vi "14_2.vi"() -> ()   [LabVIEW 2018]
uses:
  <userlib>/_OpenG.lib/dictionary/dictionary.llb/Dictionary Update (by scalar value)__ogtk.vi
panel:
  out "sum":u64
  out "Array":u64[](array[numeric])
  out "items":cluster{"key":variant, "value":variant}[](array[cluster])
  out "Mask":string[](array[string])
  out "array":string[](array[string])
  in  "Input":string
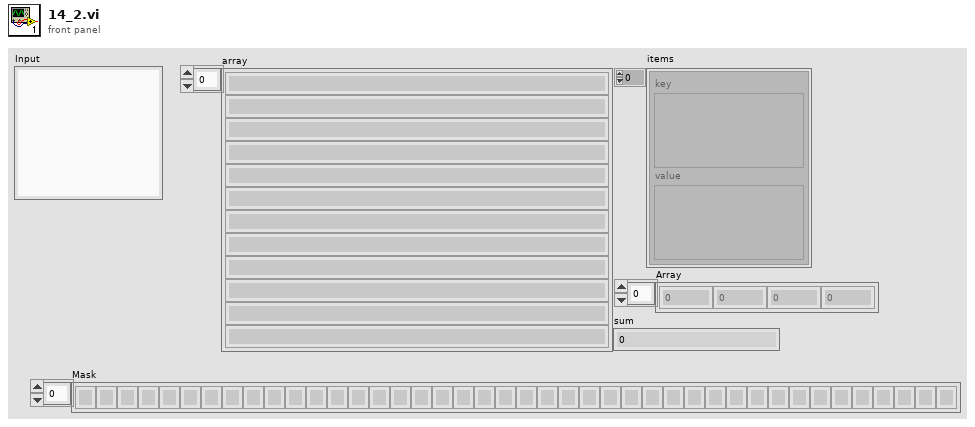
[diagram p1: front panel]
types:
  T1 = typedef "Dictionary Object RefNum__ogtk.ctl" = refnum<k1>
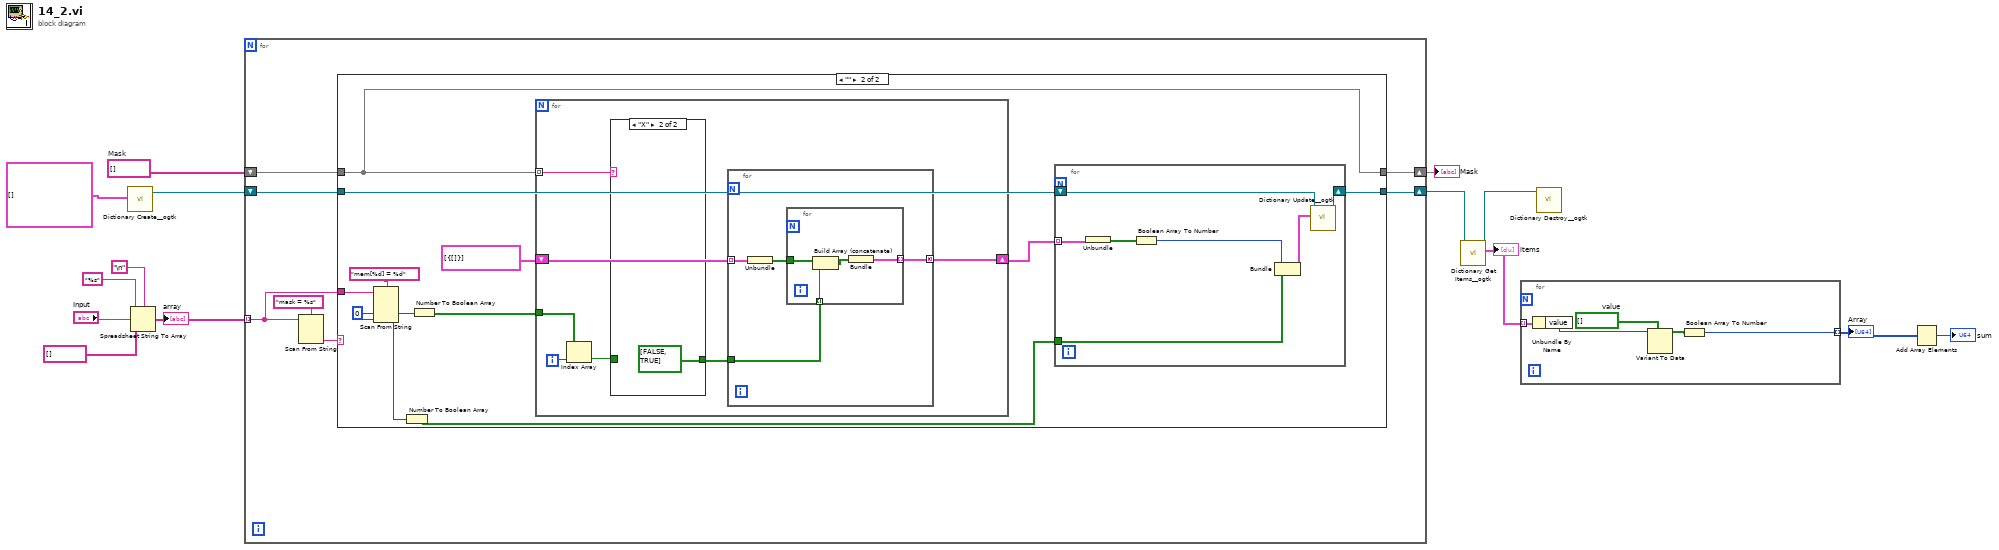
[diagram p0: block diagram]
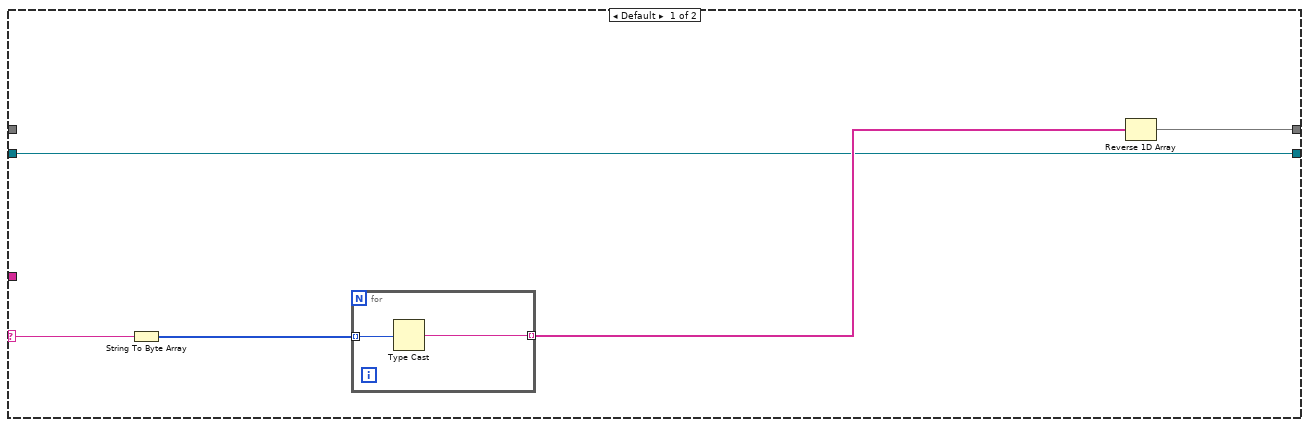
[diagram p2: hidden frame]
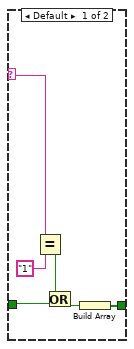
[diagram p3: hidden frame]
diagram:
  w9 = string[] []  # Mask
  n1 = call <userlib>:"Dictionary Create__ogtk.vi"("initial dictionary (empty)"=cluster{"key":u64, "value":bool[]}[] []) -> ("dictionary out"=w7:T1)  [unwired: 9 in, 1 out]
  n2 = Spreadsheet String To Array(delimiter (Tab)="\n", format string="%s", spreadsheet string="Input", array type (2D Dbl)=string[] []) -> (array=w10:string[])
  "array" <- w10
  n3 = for {
    tunnel: w10 -> [w15] mode=indexing
    shift-right: [w18] -> w8
    shift-left: w9 -> [w19]
    shift-right: [w16] -> w5
    shift-left: w7 -> [w17]
    n4 = Scan From String(format string="mask = %s", input string=w15) -> (output 1=w20:string)  [unwired: 3 in, 3 out]
    n5 = case shown="\"\"" w20 {
      selector: w20 -> [w26 _]
      tunnel: w19 -> [_ w37]
      tunnel: [w22 w37] -> w18
      tunnel: w17 -> [w23 w36]
      tunnel: [w23 w38] -> w16
      tunnel: w15 -> [_ w40]
      frame Default {
        n6 = String To Byte Array(string=w26) -> (unsigned byte array=w25:u8[])
        n7 = for {
          tunnel: w25 -> [w28] mode=indexing
          tunnel: [w27] -> w24 mode=indexing
          n8 = Type Cast(x=w28) -> (*(type *) &x=w27:string)  [unwired: 1 in]
        }
        n9 = Reverse 1D Array(array=w24) -> (reversed array=w22:string[])
      }
      frame "" {
        w33 = u64 0
        n10 = Scan From String(format string="mem[%d] = %d", input string=w40, default 1=w33, default 2=w33) -> (output 1=w32:u64, output 2=w34:u64)  [unwired: 2 in, 3 out]
        n11 = Number To Boolean Array(number=w34) -> (Boolean array=w35:bool[])
        n12 = Number To Boolean Array(number=w32) -> (Boolean array=w31:bool[])
        n13 = for {
          tunnel: w37 -> [w54] mode=indexing
          shift-right: [w48] -> w29
          shift-left: cluster{bool[]}[] [{[]}] -> [w50]
          tunnel: w31 -> [w51]
          i -> [w52]
          n14 = Index Array(array=w51, index=w52) -> (element=w53:bool)
          n15 = case shown="\"X\"" w54 {
            selector: w54 -> [w68 _]
            tunnel: [w63 bool[] [FALSE, TRUE]] -> w49
            tunnel: w53 -> [w66 _]
            frame Default {
              n16 = Equal?(x=w68, y="1") -> (x = y?=w65:bool)
              n17 = Or(x=w65, y=w66) -> (x .or. y?=w64:bool)
              n18 = Build Array(w64) -> (w63:bool[])
            }
            frame "X" {
            }
          }
          n19 = for {
            tunnel: w50 -> [w58] mode=indexing
            tunnel: w49 -> [w57]
            tunnel: [w55] -> w48 mode=concatenating
            n20 = Unbundle(w58) -> (w56:bool[])
            n21 = for {
              tunnel: w56 -> [w62]
              tunnel: w57 -> [w61] mode=indexing
              tunnel: [w59] -> w55 mode=indexing
              n22 = Build Array (concatenate)(w62, w61) -> (w60:bool[])
              n23 = Bundle(w60) -> (w59:cluster{bool[]})  [unwired: 1 in]
            }
          }
        }
        n24 = for {
          shift-right: [w47] -> w38
          shift-left: w36 -> [w45]
          tunnel: w35 -> [w44]
          tunnel: w29 -> [w42] mode=indexing
          n25 = Unbundle(w42) -> (w41:bool[])
          n26 = Boolean Array To Number(Boolean array=w41) -> (number=w43:u64)
          n27 = Bundle(w43, "Boolean array"=w44) -> (w46:cluster{u64, "Boolean array":bool[]})  [unwired: 1 in]
          n28 = call-poly <userlib>:"Dictionary Update__ogtk.vi"("key-value"=w46, "dictionary"=w45) -> ("dictionary out"=w47:T1)  [unwired: 7 in, 2 out]
        }
      }
    }
  }
  "Mask" <- w8
  n29 = call <userlib>:"Dictionary Get Items__ogtk.vi"("dictionary"=w5) -> ("items"=w3:cluster{"key":variant, "value":variant}[], "dictionary out"=w4:T1)  [unwired: 8 in, 1 out]
  "items" <- w3
  n30 = for {
    tunnel: w3 -> [w74] mode=indexing
    tunnel: [w70] -> w2 mode=indexing
    w73 = bool[] []  # value
    n31 = Unbundle By Name(w74) -> ("value"=w72:variant)
    n32 = Variant To Data(type=w73, Variant=w72) -> (data=w71:bool[])  [unwired: 1 in, 1 out]
    n33 = Boolean Array To Number(Boolean array=w71) -> (number=w70:u64)
  }
  "Array" <- w2
  n34 = call <userlib>:"Dictionary Destroy__ogtk.vi"("dictionary"=w4) -> ()  [unwired: 10 in, 1 out]
  n35 = Add Array Elements(numeric array=w2) -> (sum=→"sum":u64)
